vi "S2DS_Read external instrument.vi"(7 "error in (no error)":errorcluster, 10 "Instrument parameters":T1) -> (0 "error out":errorcluster, 2 "data out":dbl[](array[numeric]), 3 "Instrument parameters out":T1)   [LabVIEW 2025]
uses:
  TYPE DEFS/S2DS_Instrument parameters.ctl
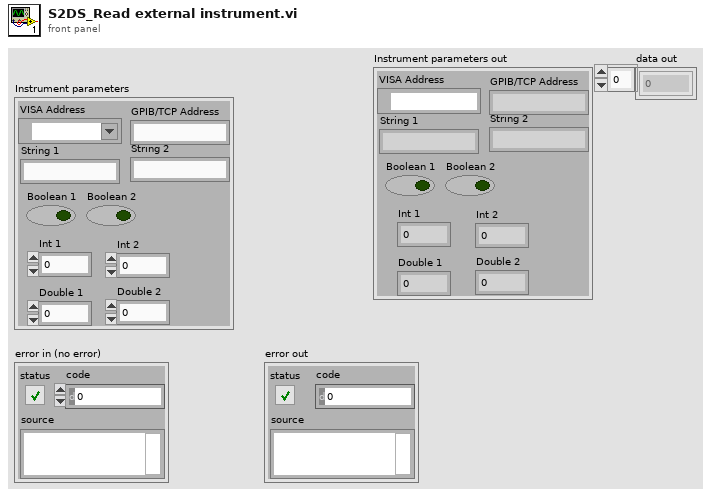
[diagram p1: front panel]
types:
  T1 = typedef "S2DS_Instrument parameters.ctl" = cluster{"VISA Address":refnum<visa-resource-name>, "GPIB/TCP Address":string, "String 1":string, "String 2":string, "Boolean 1":bool, "Boolean 2":bool, "Int 1":i32, "Int 2":i32, "Double 1":dbl, "Double 2":dbl}
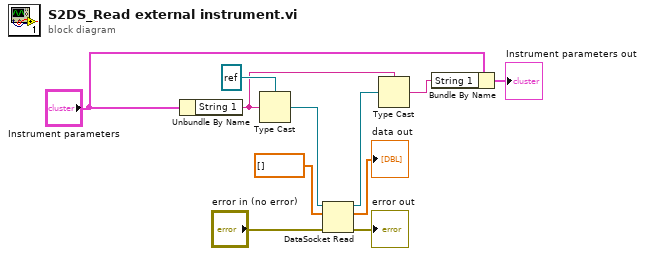
[diagram p0: block diagram]
diagram:
  n1 = Unbundle By Name("Instrument parameters") -> ("String 1"=w6:string)
  n2 = Type Cast(type=refnum<k13> refnum ("connection id"), x=w6) -> (*(type *) &x=w9:refnum<k13>)
  n3 = DataSocket Read(8:"error in (no error)", 10:dbl[] [], 11:w9) -> (0:→"error out":errorcluster, 2:→"data out":dbl[], 3:w7:refnum<k13>)  [unwired: 2 in, 4 out]
  n4 = Type Cast(type=w6, x=w7) -> (*(type *) &x=w5:string)
  n5 = Bundle By Name(cluster="Instrument parameters", "String 1"=w5) -> (→"Instrument parameters out":T1)
